vi "Read Collimation data.vi"(8 "error in (no error)":errorcluster, 11 "Fiber Auto Collimation state data in":refnum<class "Fiber Auto Collimation state data.lvclass">) -> (0 "error out":errorcluster, 2 "BV Data":T1={"Centroid X[um]"=nan, "Centroid Y[um]"=nan, "PeakResp.[%]"=nan, "Knife Edge X[mm]"=nan, "Knife Edge Y[mm]"=nan, "Circularity"=nan, "Collimation Result"=FALSE} {"PeakResp.[%]" format="%.0g"}, 3 "Fiber Auto Collimation state data out":refnum<class "Fiber Auto Collimation state data.lvclass">)   [LabVIEW 2018, in "Fiber Auto Collimation state data.lvclass"]
doc: "This \"LIV test data\" is just a placeholder and example for how real test data might be stored. This accessor plus its data in the state data class private control probably need to be removed or replaced with something to hold test data for the actual station."
uses:
  Fiber Auto Collimation state data.lvclass
  BV Data.ctl
  Fiber Auto Collimation state data.lvclass/Fiber Auto Collimation state data.ctl
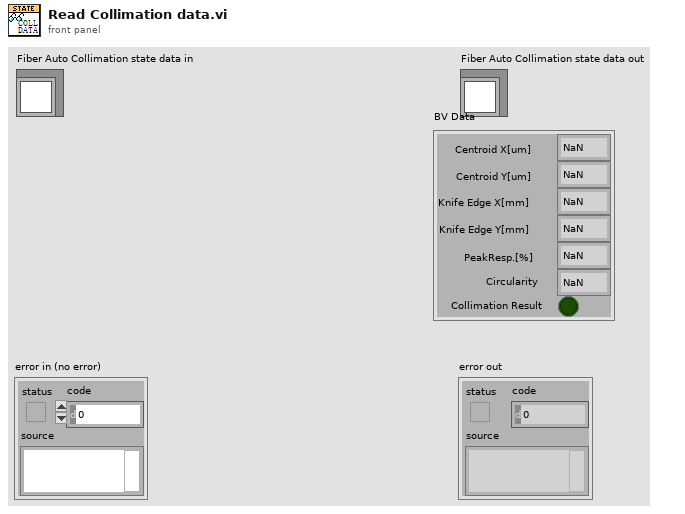
[diagram p1: front panel]
types:
  T1 = typedef "Fiber Auto Collimation state data.lvclass/BV Data.ctl" = cluster{"Centroid X[um]":sgl, "Centroid Y[um]":sgl, "PeakResp.[%]":dbl, "Knife Edge X[mm]":sgl, "Knife Edge Y[mm]":sgl, "Circularity":sgl, "Collimation Result":bool}
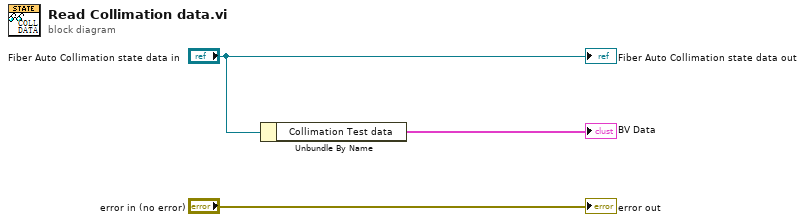
[diagram p0: block diagram]
diagram:
  n1 = Unbundle By Name("Fiber Auto Collimation state data in") -> ("Collimation Test data"=→"BV Data":T1)
  "error out" <- "error in (no error)"
  "Fiber Auto Collimation state data out" <- "Fiber Auto Collimation state data in"
